vi "Path Root SLM.vi"(0 "VI Ref IN":refnum<vi>) -> (4 "VI Ref OUT":refnum<vi>)   [LabVIEW 2014]
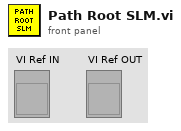
[diagram p1: front panel]
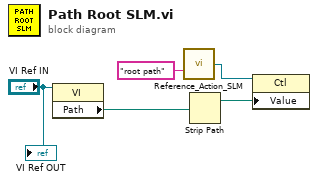
[diagram p0: block diagram]
diagram:
  n1 = property class="VI"(reference="VI Ref IN") -> ("Path"=w2:path)  [unwired: 1 in, 2 out]
  n2 = call "Reference_Action_SLM.vi"("Control Name"="root path") -> ("Ref OUT"=w3:refnum<vi>)  [unwired: 12 in, 2 out]
  n3 = Strip Path(path=w2) -> (stripped path=w1:path)  [unwired: 1 out]
  n4 = property class="Ctl"(reference=w3, "Value"=w1) -> ()  [unwired: 1 in, 2 out]
  "VI Ref OUT" <- "VI Ref IN"
